vi "Recieve Timer Tick.vi"(8 "error in (no error)":errorcluster, 10 "Time Stamp Control":timestamp, 11 "Mag Lab Measurement in":refnum<class "Mag Lab Measurement.lvclass">) -> (0 "error out":errorcluster, 3 "Mag Lab Measurement out":refnum<class "Mag Lab Measurement.lvclass">)   [LabVIEW 2015, in "Mag Lab Measurement.lvclass"]
uses:
  Mag Lab Measurement.lvclass
  Mag Lab Measurement.lvclass/Mag Lab Measurement.ctl
  <vilib>/ActorFramework/Actor/Actor.lvclass/Actor.ctl
  <vilib>/ActorFramework/Message Enqueuer/Message Enqueuer.lvclass/Message Enqueuer.ctl
  <vilib>/ActorFramework/Message Enqueuer/Init from Existing Queue.vi
  <vilib>/ActorFramework/Message Enqueuer/Enqueue.vi
  <vilib>/ActorFramework/Message Priority Queue/Priority Enqueue.vi
  Mag Lab Measure Base/Mag Lab Measure Base.lvclass
  <vilib>/ActorFramework/Message Enqueuer/Message Enqueuer.lvclass
  Mag Lab Measurement Messages/Acquire Result Msg/Acquire Result Msg.lvclass
  <vilib>/ActorFramework/Actor/Actor.lvclass
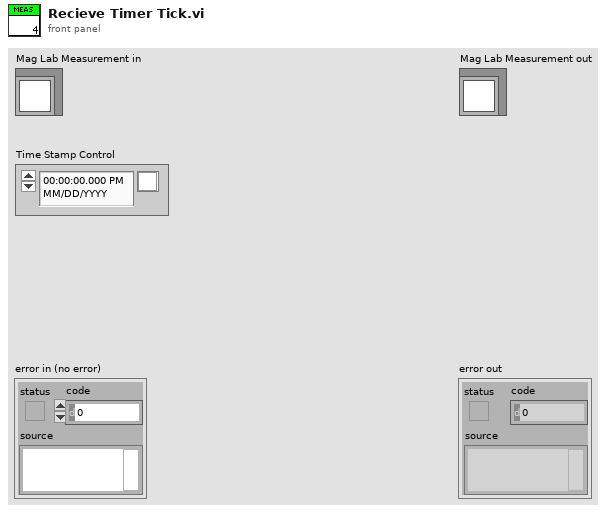
[diagram p1: front panel]
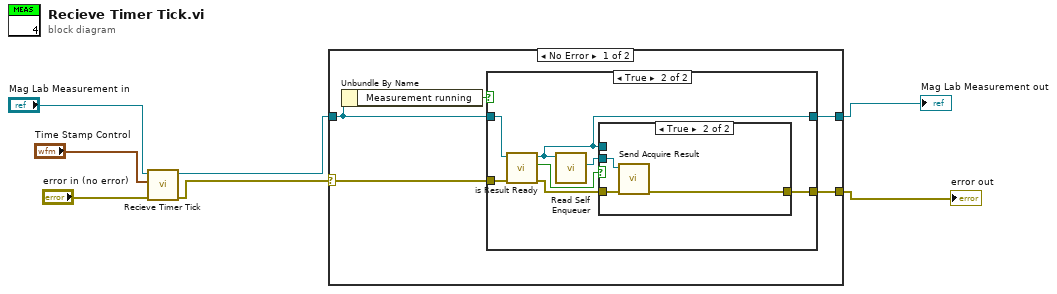
[diagram p0: block diagram]
diagram:
  n1 = call-parent "Recieve Timer Tick.vi"("error in (no error)"="error in (no error)", "Time Stamp Control"="Time Stamp Control", "Mag Lab Measure Base in"="Mag Lab Measurement in") -> ("error out"=w3:errorcluster, "Mag Lab Measure Base out"=w4:refnum<class "Mag Lab Measurement.lvclass">)  [unwired: 7 in]
  n2 = case shown="No Error" w3 {
    selector: w3 -> [w11 w27]
    tunnel: [w10 w27] -> w2
    tunnel: [w12 w26] -> w1
    tunnel: w4 -> [w9 w26]
    frame No Error {
      n3 = Unbundle By Name(w9) -> ("Measurement running"=w8:bool)
      n4 = case shown="True" w8 {
        tunnel: w9 -> [w13 w21]
        tunnel: [w13 w18] -> w12
        tunnel: w11 -> [w14 w17]
        tunnel: [w14 w15] -> w10
        frame False {
        }
        frame True {
          n5 = call-dynamic "is Result Ready.vi"("error in (no error)"=w17, "Mag Lab Measurement in"=w21) -> ("error out"=w16:errorcluster, "Result Available"=w20:bool, "Mag Lab Measurement out"=w18:refnum<class "Mag Lab Measurement.lvclass">)  [unwired: 7 in]
          n6 = call <vilib>:"Read Self Enqueuer.vi"("Actor"=w18) -> ("Self Enqueuer"=w19:refnum<class "Message Enqueuer.lvclass">)  [unwired: 10 in]
          n7 = case shown="True" w20 {
            tunnel: w19 -> [_ w25]
            tunnel: w18 -> [_ _]
            tunnel: w16 -> [w22 w24]
            tunnel: [w22 w23] -> w15
            frame False {
            }
            frame True {
              n8 = call "Send Acquire Result.vi"("error in (no error)"=w24, "Message Enqueuer"=w25) -> ("error out"=w23:errorcluster)  [unwired: 8 in, 1 out]
            }
          }
        }
      }
    }
    frame Error {
    }
  }
  "error out" <- w2
  "Mag Lab Measurement out" <- w1
